vi "case_select.vi"() -> ()   [LabVIEW 2017]
panel:
  in  "Output selection":string(combo)
  out "Converted value":string
  out "?":bool
  out "?":bool
  out "?":bool
  out "?":bool
  out "?":bool
  out "?":bool
  out "?":bool
  out "?":bool
  in  "Binary Input":bool[](array[boolean])
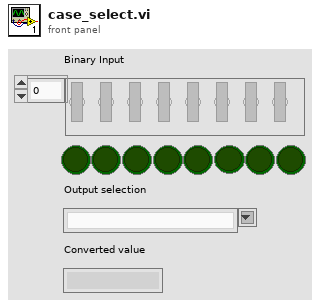
[diagram p1: front panel]
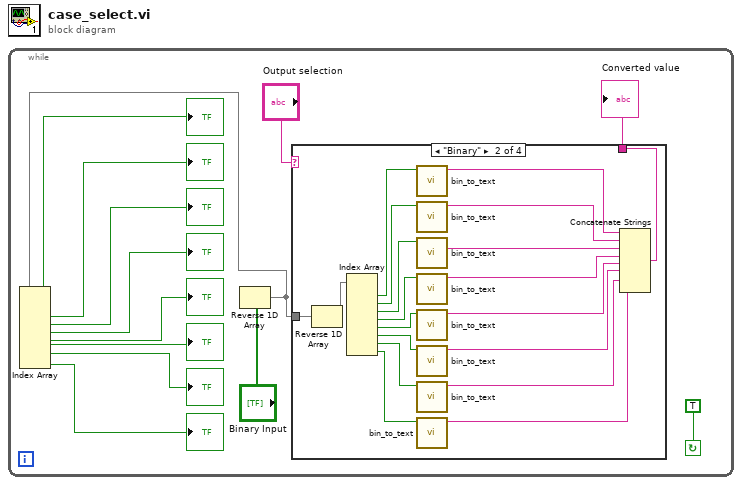
[diagram p0: block diagram]
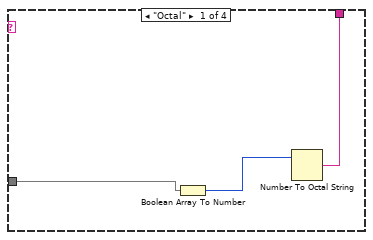
[diagram p2: hidden frame]
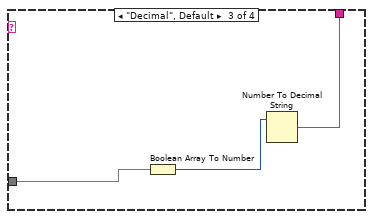
[diagram p3: hidden frame]
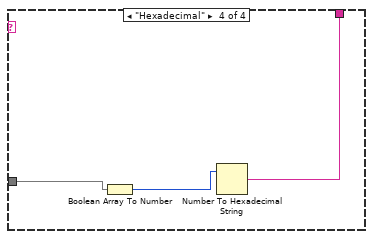
[diagram p4: hidden frame]
diagram:
  n1 = while {
    stop <- TRUE continue-if-true
    n2 = Reverse 1D Array(array="Binary Input") -> (reversed array=w1:bool[])
    n3 = Index Array(array=w1) -> (element #1=→"?":bool, element #2=→"?":bool, element #3=→"?":bool, element #4=→"?":bool, element #5=→"?":bool, element #6=→"?":bool, element #7=→"?":bool, element #8=→"?":bool)  [unwired: 8 in]
    n4 = case shown="\"Binary\"" "Output selection" {
      tunnel: [w15 w35 w37 w40] -> w4
      tunnel: w1 -> [w16 w17 w38 w41]
      frame "Octal" {
        n5 = Boolean Array To Number(Boolean array=w16) -> (number=w14:u32)
        n6 = Number To Octal String(2:w14) -> (0:w15:string)  [unwired: 1 in]
      }
      frame "Binary" {
        n7 = Reverse 1D Array(array=w17) -> (reversed array=w18:bool[])
        n8 = Index Array(array=w18) -> (element #1=w34:bool, element #2=w33:bool, element #3=w32:bool, element #4=w31:bool, element #5=w30:bool, element #6=w29:bool, element #7=w28:bool, element #8=w27:bool)  [unwired: 8 in]
        n9 = call "bin_to_text.vi"("Boolean in"=w34) -> ("String"=w26:string)  [unwired: 10 in]
        n10 = call "bin_to_text.vi"("Boolean in"=w33) -> ("String"=w25:string)  [unwired: 10 in]
        n11 = call "bin_to_text.vi"("Boolean in"=w32) -> ("String"=w24:string)  [unwired: 10 in]
        n12 = call "bin_to_text.vi"("Boolean in"=w31) -> ("String"=w23:string)  [unwired: 10 in]
        n13 = call "bin_to_text.vi"("Boolean in"=w30) -> ("String"=w22:string)  [unwired: 10 in]
        n14 = call "bin_to_text.vi"("Boolean in"=w29) -> ("String"=w21:string)  [unwired: 10 in]
        n15 = call "bin_to_text.vi"("Boolean in"=w28) -> ("String"=w20:string)  [unwired: 10 in]
        n16 = call "bin_to_text.vi"("Boolean in"=w27) -> ("String"=w19:string)  [unwired: 10 in]
        n17 = Concatenate Strings(w26, w25, w24, w23, w22, w21, w20, w19) -> (w35:string)
      }
      frame "Decimal", Default {
        n18 = Boolean Array To Number(Boolean array=w38) -> (number=w36:u32)
        n19 = Number To Decimal String(number=w36) -> (decimal integer string=w37:string)  [unwired: 1 in]
      }
      frame "Hexadecimal" {
        n20 = Boolean Array To Number(Boolean array=w41) -> (number=w39:u32)
        n21 = Number To Hexadecimal String(2:w39) -> (0:w40:string)  [unwired: 1 in]
      }
    }
    "Converted value" <- w4
  }
